vi "parseString.vi"(8 "error in (no error)":errorcluster, 10 "stringCommand":string, 11 "CommandParser in":refnum<class "CommandParser.lvclass">) -> (0 "error out":errorcluster, 1 "parameter":variant, 2 "monoCommand":T1, 3 "CommandParser out":refnum<class "CommandParser.lvclass">)   [LabVIEW 2016, in "CommandParser.lvclass"]
uses:
  CommandParser.lvclass
  Typedefs/MonoCommand.ctl
  Typedefs/wavelength.ctl
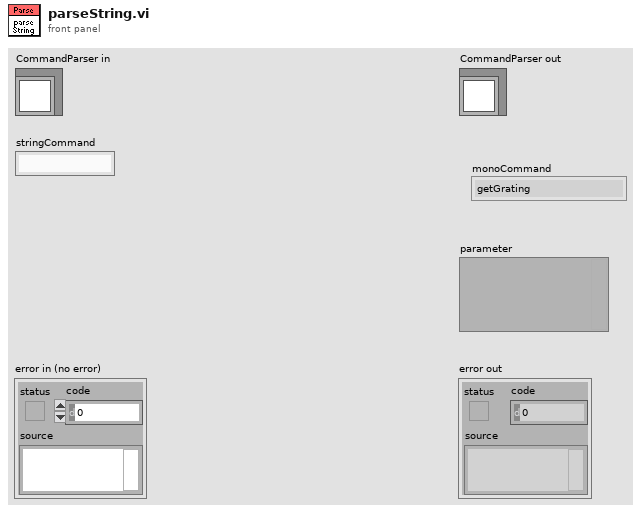
[diagram p1: front panel]
types:
  T1 = typedef "MonoCommand.ctl" = enum16{"getGrating", "getFrontEntranceSlitPosition", "getFrontExitSlitPosition", "getWavelength", "setWavelength", "setGrating", "setFrontEntranceSlitPosition", "setFrontExitSlitPosition", "calibrateWavelength", "getStatus", "Unknown", "reset", "setAll"}
  T2 = typedef "wavelength.ctl" = dbl
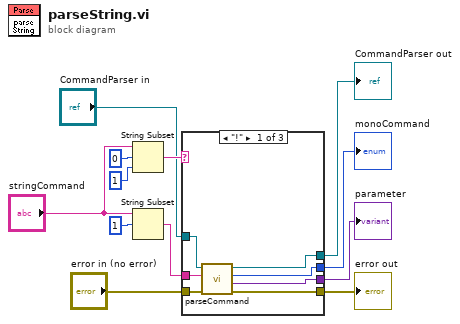
[diagram p0: block diagram]
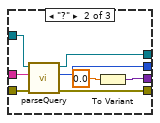
[diagram p2: hidden frame]
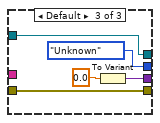
[diagram p3: hidden frame]
diagram:
  n1 = String Subset(string="stringCommand", offset (0)=0, length (rest)=1 ("length (len. of substring)")) -> (substring=w10:string)
  n2 = String Subset(string="stringCommand", offset (0)=1) -> (substring=w1:string)  [unwired: 1 in]
  n3 = case shown="\"!\"" w10 {
    tunnel: [w15 w24 MonoCommand."Unknown" ("monoCommand")] -> w9
    tunnel: "CommandParser in" -> [w19 w27 w31]
    tunnel: [w18 w23 w31] -> w7
    tunnel: "error in (no error)" -> [w17 w26 w30]
    tunnel: [w16 w25 w30] -> w5
    tunnel: [w14 w21 w28] -> w4
    tunnel: w1 -> [w13 w20 _]
    frame "!" {
      n4 = call "parseCommand.vi"("error in (no error)"=w17, "CMDString"=w13, "CommandParser in"=w19) -> ("error out"=w16:errorcluster, "parameter"=w14:variant, "MonoCommand"=w15:T1, "CommandParser out"=w18:refnum<class "CommandParser.lvclass">)  [unwired: 5 in]
    }
    frame "?" {
      n5 = call "parseQuery.vi"("error in (no error)"=w26, "QueryString"=w20, "CommandParser in"=w27) -> ("error out"=w25:errorcluster, "MonoCommand"=w24:T1, "CommandParser out"=w23:refnum<class "CommandParser.lvclass">)  [unwired: 6 in]
      n6 = To Variant(anything=T2 0.0 ("wavelength")) -> (Variant=w21:variant)
    }
    frame Default {
      n7 = To Variant(anything=T2 0.0 ("wavelength")) -> (Variant=w28:variant)
    }
  }
  "error out" <- w5
  "CommandParser out" <- w7
  "monoCommand" <- w9
  "parameter" <- w4
